vi "Read Template.vi"(8 "error in (no error)":errorcluster, 11 "CHEAH in":refnum<class "CHEAH.lvclass">) -> (0 "error out":errorcluster, 2 "Template":string, 3 "CHEAH out":refnum<class "CHEAH.lvclass">)   [LabVIEW 2021, in "_Template.lvlib" / "CHEAH.lvclass"]
uses:
  CHEAH.lvclass
  CHEAH.lvclass/CHEAH.ctl
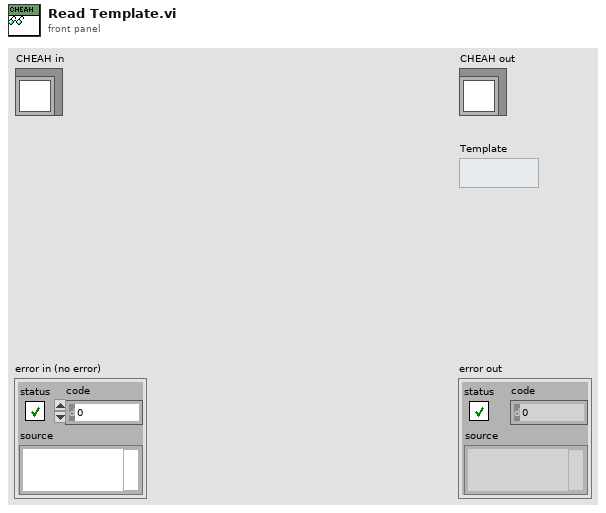
[diagram p1: front panel]
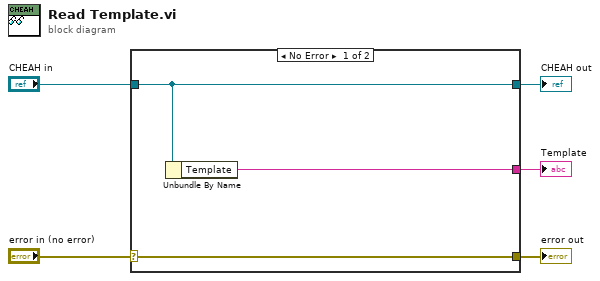
[diagram p0: block diagram]
diagram:
  n1 = case shown="No Error" "error in (no error)" {
    selector: "error in (no error)" -> [w8 w9]
    tunnel: [w8 w9] -> w4
    tunnel: [w7 w10] -> w2
    tunnel: "CHEAH in" -> [w7 w10]
    tunnel: [w6 _] -> w1
    frame No Error {
      n2 = Unbundle By Name(w7) -> ("Template"=w6:string)
    }
    frame Error {
    }
  }
  "error out" <- w4
  "CHEAH out" <- w2
  "Template" <- w1
